vi "GetWaveformInfoArray.vi"(8 "error in (no error)":errorcluster, 11 "TektronixDPOSimple in":refnum<class "Tektronix MDO MSO DPO.lvclass">) -> (0 "error out":errorcluster, 3 "TektronixDPOSimple out":refnum<class "Tektronix MDO MSO DPO.lvclass">)   [LabVIEW 2020, in "Tektronix MDO MSO DPO.lvclass"]
doc: "Read the Waveform Info from the physical device"
uses:
  Tektronix MDO MSO DPO.lvclass
  Tektronix MDO MSO DPO.lvclass/Tektronix MDO MSO DPO.ctl
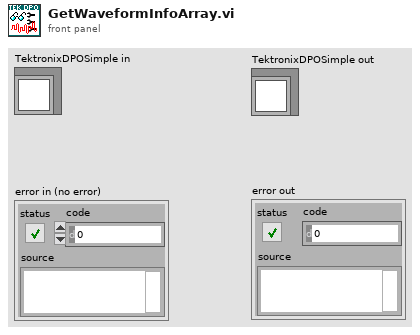
[diagram p1: front panel]
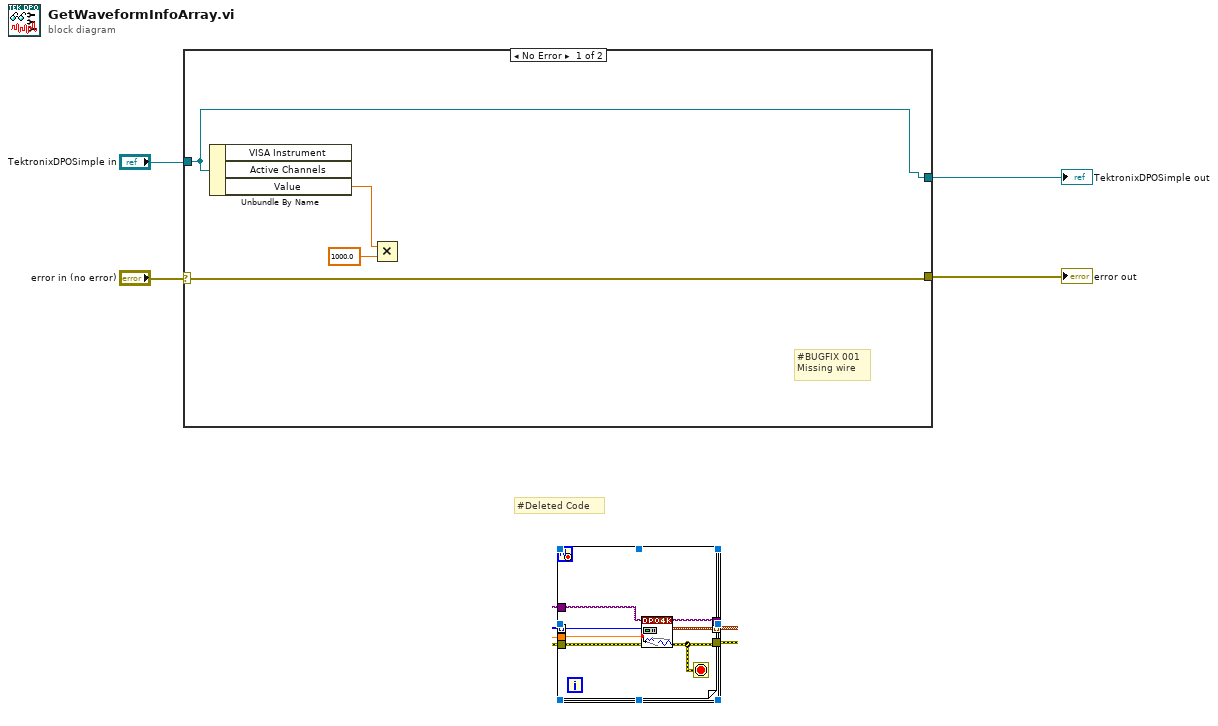
[diagram p0: block diagram]
diagram:
  # "#Deleted Code"
  n1 = case shown="No Error" "error in (no error)" {
    selector: "error in (no error)" -> [w6 w10]
    tunnel: "TektronixDPOSimple in" -> [w5 w9]
    tunnel: [w6 w10] -> w3
    tunnel: [w5 w9] -> w1
    frame No Error {
      # "#BUGFIX 001\nMissing wire"
      n2 = Unbundle By Name(w5) -> ("Value"=w8:dbl)  [unwired: 2 out]
      n3 = Multiply(x=w8, y=1000.0) -> ()  [unwired: 1 out]
    }
    frame Error {
    }
  }
  "error out" <- w3
  "TektronixDPOSimple out" <- w1
